vi "Multipart Upload.vi"() -> ()   [LabVIEW 2020]
uses:
  datasources/dataset/dataset.lvclass
  nominal types/channelConfig/channelConfig.lvclass
  Nominal Client.lvclass/Nominal Client.ctl
  nominal types/workspace/workspace.lvclass/workspace.ctl
  0bc17519-4080-4d35-abf7-1c68a97f5e00.vi
  4f2f9e19-0aaf-42d0-b22f-a8130bfdc877.vi
  private_data.set.vi
  nominal types/workspace/rid.get.vi
  nominal types/workspace/id.get.vi
  <vilib>/AdvancedString/1D String Array to Delimited String.vi
  workspace.set.vi
  nominal types/timestampManifest/noManifest/noManifest.lvclass
  C:/code/labview-client/lv_src/nominal types/timestampManifest/timestampManifest/timestampManifest.lvclass
  datasources/s3/s3.lvclass
  C:/code/labview-client/lv_src/datasources/source/source.lvclass
  <vilib>/Utility/file.llb/Application Directory.vi
  <vilib>/Utility/error.llb/Error Cluster From Error Code.vi
  Palette Items/who_am_i.vi
  workspace_cache.get_from_rid.vi
  workspace_cache.get.vi
  datasources/source/create_s3.vi
  datasources/target/create_new.vi
  nominal types/timestampManifest/create.noManifest_scale_factor.vi
  ingest_video.vi
  video.get_ingest_status.vi
  User/User.lvclass
  Nominal Client.lvclass
  nominal types/workspace/workspace.lvclass
  submodules/reqwest-labview/lv-src/reqwest/reqwest.lvclass
  Nominal Client MultiPart Upload/Multipart Upload.lvclass
  datasources/source/source.lvclass
  nominal types/timestampManifest/timestampManifest.lvlib
  datasources/target/target.lvclass
  nominal types/properties/properties.lvclass
  C:/code/labview-client/lv_src/datasources/payload/payload.lvclass
  C:/code/labview-client/lv_src/nominal types/timestampManifest/noManifest/noManifest.lvclass
  C:/code/labview-client/lv_src/datasources/s3/s3.lvclass
panel:
  out "Ingest Progress":dbl(slide) scale=0.0..1.0
  in  "Description":string
  in  "Title":string
  in  "Stop wait":bool
  in  "File Path":path
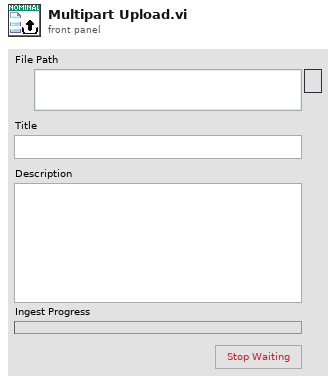
[diagram p1: front panel]
types:
  T1 = cluster{"dataset":refnum<class "dataset.lvclass">, "channelConfig":refnum<class "channelConfig.lvclass">}
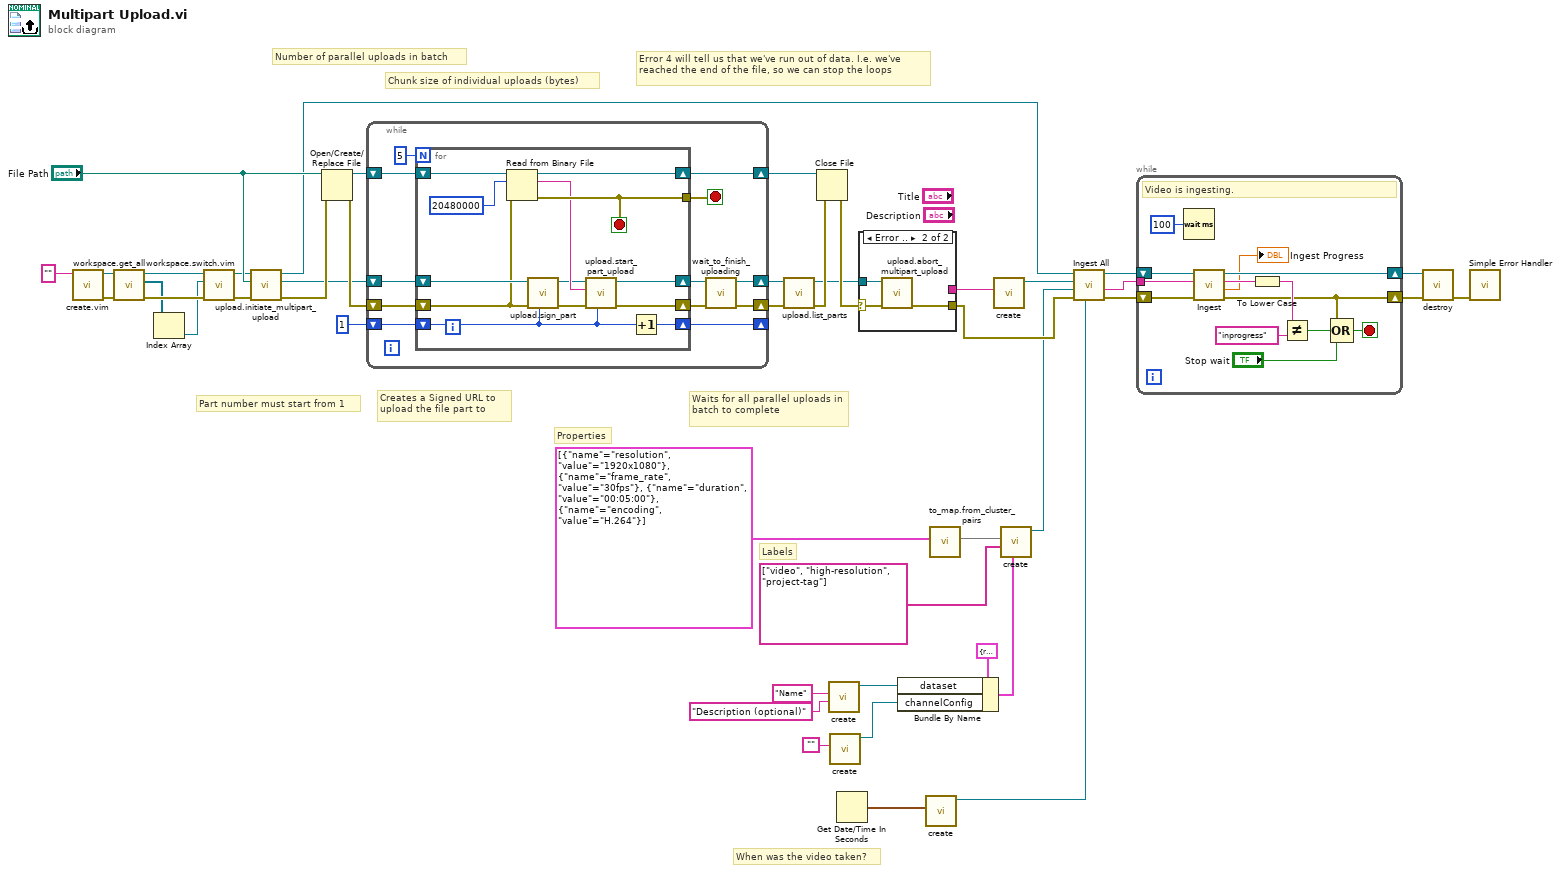
[diagram p0: block diagram]
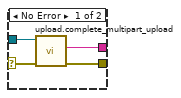
[diagram p2: hidden frame]
diagram:
  # "When was the video taken?"
  # "Waits for all parallel uploads in batch to complete"
  # "Creates a Signed URL to upload the file part to"
  # "Chunk size of individual uploads (bytes)"
  # "Number of parallel uploads in batch"
  # "Part number must start from 1"
  # "Error 4 will tell us that we've run out of data. I.e. we've reached the end of the file, so we can stop the loops"
  # "Labels"
  # "Properties"
  n1 = call "create.vim"("API Token (string or path)"="") -> ("error out"=w11:errorcluster, "Nominal Client"=w12:refnum<class "Nominal Client.lvclass">)  [unwired: 8 in, 1 out]
  n2 = call "workspace.get_all.vi"("error in"=w11, "Nominal Client in"=w12) -> ("error out"=w10:errorcluster, "Workspaces"=w6:refnum<class "workspace.lvclass">[], "Nominal Client out"=w7:refnum<class "Nominal Client.lvclass">)  [unwired: 7 in]
  n3 = Index Array(array=w6) -> (element=w5:refnum<class "workspace.lvclass">)  [unwired: 1 in]
  n4 = call "workspace.switch.vim"("error in"=w10, "Workspace (Object, RID, Path)"=w5, "Nominal Client in"=w7) -> ("error out"=w9:errorcluster, "Nominal Client out"=w8:refnum<class "Nominal Client.lvclass">)  [unwired: 7 in]
  n5 = call "upload.initiate_multipart_upload.vi"("error in"=w9, "File Path"="File Path", "Nominal Client in"=w8) -> ("error out"=w34:errorcluster, "Multipart Upload"=w32:refnum<class "Multipart Upload.lvclass">, "Nominal Client out"=w24:refnum<class "Nominal Client.lvclass">)  [unwired: 6 in]
  n6 = Open/Create/Replace File(file path (use dialog)="File Path", error in=w34) -> (refnum out=w38:refnum<file>, error out=w33:errorcluster)  [unwired: 4 in, 1 out]
  n7 = while {
    shift-right: [w45] -> w40
    shift-left: w32 -> [w56]
    shift-right: [w48] -> w35
    shift-left: w33 -> [w50]
    shift-right: [w54] -> _
    shift-left: 1 -> [w55]
    shift-right: [w51] -> w37
    shift-left: w38 -> [w53]
    stop <- w52 stop-if-true
    n8 = for {
      N: 5 -> [_]
      shift-right: [w59] -> w46
      shift-left: w56 -> [w69]
      shift-right: [w68] -> w54
      shift-left: w55 -> [w58]
      tunnel: [w64] -> w52
      shift-right: [w65] -> w51
      shift-left: w53 -> [w66]
      shift-right: [w62] -> w49
      shift-left: w50 -> [w57]
      stop <- w64 stop-if-true
      n9 = Read from Binary File(8:w57, 10:20480000 ("count (1)"), 11:w66) -> (0:w64:errorcluster, 2:w61:string, 3:w65:refnum<file>)  [unwired: 3 in, 1 out]
      n10 = call "upload.sign_part.vi"("Part Number"=w58, "error in"=w57, "Multipart Upload in"=w69) -> ("error out"=w63:errorcluster, "Multipart Upload out"=w60:refnum<class "Multipart Upload.lvclass">)  [unwired: 7 in]
      n11 = call "upload.start_part_upload.vi"("Part Number"=w58, "error in"=w63, "File Part Binary"=w61, "Multipart Upload"=w60) -> ("error out"=w62:errorcluster, "Multipart Upload out"=w59:refnum<class "Multipart Upload.lvclass">)  [unwired: 6 in]
      n12 = Increment(x=w58) -> (x+1=w68:i32)
    }
    n13 = call "wait_to_finish_uploading.vi"("error in"=w49, "Multipart Upload in"=w46) -> ("error out"=w48:errorcluster, "Multipart Upload out"=w45:refnum<class "Multipart Upload.lvclass">)  [unwired: 8 in]
  }
  n14 = call "upload.list_parts.vi"("error in"=w35, "Multipart Upload"=w40) -> ("error out"=w31:errorcluster, "Multipart Upload out"=w29:refnum<class "Multipart Upload.lvclass">)  [unwired: 8 in]
  n15 = Close File(refnum=w37, error in=w31) -> (error out=w30:errorcluster)  [unwired: 1 out]
  n16 = call "create.vi"("Description"="Description (optional)", "Name"="Name") -> ("dataset"=w18:refnum<class "dataset.lvclass">)  [unwired: 9 in]
  n17 = call "create.vi"("prefixTreeDelimiter"="") -> ("channelConfig"=w14:refnum<class "channelConfig.lvclass">)  [unwired: 10 in]
  n18 = Get Date/Time In Seconds() -> (seconds since 1Jan1904=w25:timestamp)
  n19 = case shown="Error .." w30 {
    selector: w30 -> [w71 w76]
    tunnel: [w73 _] -> w27
    tunnel: w29 -> [w72 w75]
    tunnel: [w70 w74] -> w23
    frame No Error {
      n20 = call "upload.complete_multipart_upload.vi"("error in"=w71, "Multipart Upload in"=w72) -> ("error out"=w70:errorcluster, "S3 Path to File"=w73:string)  [unwired: 8 in]
    }
    frame Error {
      n21 = call "upload.abort_multipart_upload.vi"("error in"=w76, "Multipart Upload"=w75) -> ("error out"=w74:errorcluster)  [unwired: 9 in]
    }
  }
  n22 = Bundle By Name(cluster=T1 {"dataset"=refnum, "channelConfig"=refnum} ("Optional"), "dataset"=w18, "channelConfig"=w14) -> (w17:T1)
  n23 = call-poly "create.vi"("startingTimestamp"=w25) -> ("Timestamp Manifest"=w4:refnum<class "noManifest.lvclass">)  [unwired: 10 in]
  n24 = call "to_map.from_cluster_pairs.vi"("properties (cluster pairs)"=cluster{"name":string, "value":string}[] [{"name"="resolution", "value"="1920x1080"}, {"name"="frame_rate", "value"="30fps"}, {"name"="duration", "value"="00:05:00"}, {"name"="encoding", "value"="H.264"}] ("properties")) -> ("properties (map)"=w1:map{string, string})  [unwired: 10 in]
  n25 = call-poly "create.vi"("Path"=w27) -> ("source"=w28:refnum<class "s3.lvclass">)  [unwired: 10 in]
  n26 = call-poly "create.vi"("Optional"=w17, "Labels"=string[] ["video", "high-resolution", "project-tag"], "Properties"=w1) -> ("New Target"=w20:refnum<class "target.lvclass">)  [unwired: 8 in]
  n27 = call-poly "Ingest All.vi"("Timestamp Manifest"=w4, "error in"=w23, "Target"=w20, "Source"=w28, "Nominal Client in"=w24) -> ("error out"=w22:errorcluster, "videoFileRid"=w26:string, "Nominal Client out"=w21:refnum<class "Nominal Client.lvclass">)  [unwired: 3 in, 1 out]
  n28 = while {
    shift-right: [w87] -> w43
    shift-left: w21 -> [w89]
    shift-right: [w84] -> w42
    shift-left: w22 -> [w88]
    tunnel: w26 -> [w78]
    stop <- w81 stop-if-true
    # "Video is ingesting."
    n29 = Wait (ms)(milliseconds to wait=u32 100) -> ()  [unwired: 1 out]
    n30 = call-poly "Ingest.vi"("error in"=w88, "Video RID"=w78, "Nominal Client in"=w89) -> ("error out"=w84:errorcluster, "Progress (0-1)"=→"Ingest Progress":dbl, "Status"=w80:string, "Nominal Client out"=w87:refnum<class "Nominal Client.lvclass">)  [unwired: 5 in]
    n31 = To Lower Case(string=w80) -> (all lower case string=w85:string)
    n32 = Not Equal?(x=w85, y="inprogress") -> (x != y?=w83:bool)
    n33 = Compound Arithmetic op=OR(w84, w83, "Stop wait") -> (w81:bool)
  }
  n34 = call "destroy.vi"("error in"=w42, "Nominal Client"=w43) -> ("error out"=w44:errorcluster)  [unwired: 9 in]
  n35 = call <vilib>:"Simple Error Handler.vi"("error in (no error)"=w44) -> ()  [unwired: 4 in, 5 out]
